vi "Send Encoder Values to Dashboard.vi"(1 "Encoder Value":dbl, 2 "wheel diameteres":dbl, 3 "Endcoder Name":string="Numeric Array") -> ()   [LabVIEW 2013]
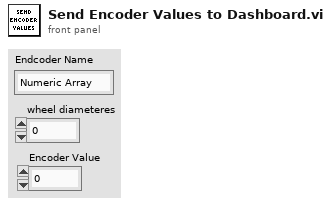
[diagram p1: front panel]
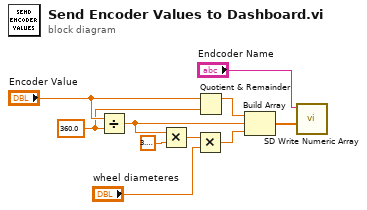
[diagram p0: block diagram]
diagram:
  w6 = 360.0 ("y")
  n1 = Divide(x="Encoder Value", y=w6) -> (x/y=w2:dbl)
  n2 = Multiply(x=w2, y=3.141592653589793) -> (x*y=w8:dbl)
  n3 = Multiply(x=w8, y="wheel diameteres") -> (x*y=w1:dbl)
  n4 = Quotient & Remainder(x="Encoder Value", y=w6) -> (x-y*floor(x/y)=w3:dbl)  [unwired: 1 out]
  n5 = Build Array(w3, w2, w1) -> (w4:dbl[])
  n6 = call <vilib>:"SD Write Numeric Array.vi"("Numeric Array"=w4, "Name"="Endcoder Name") -> ()  [unwired: 8 in, 2 out]
